vi "zs_newexample.vi"() -> ()   [LabVIEW 2014]
uses:
  <vilib>/regexp/Match Regular Expression.xnode
panel:
  out "错误输出":errorcluster
  out "数据输出":string
  out "standard error":string caption="标准错误"
  out "error out":errorcluster caption="错误输出"
  out "数组":string[][](array[string])
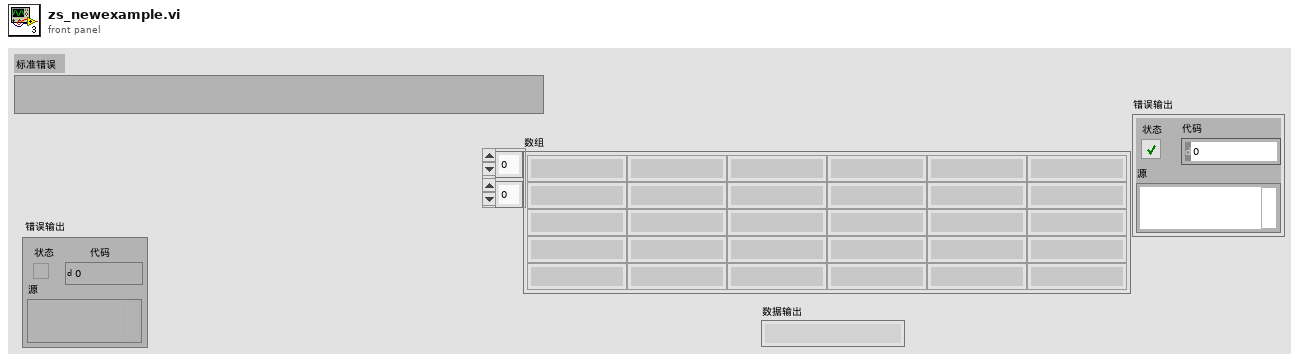
[diagram p1: front panel]
types:
  T1 = enum16{"Standard", "Buffered", "CRLF", "Immediate"}
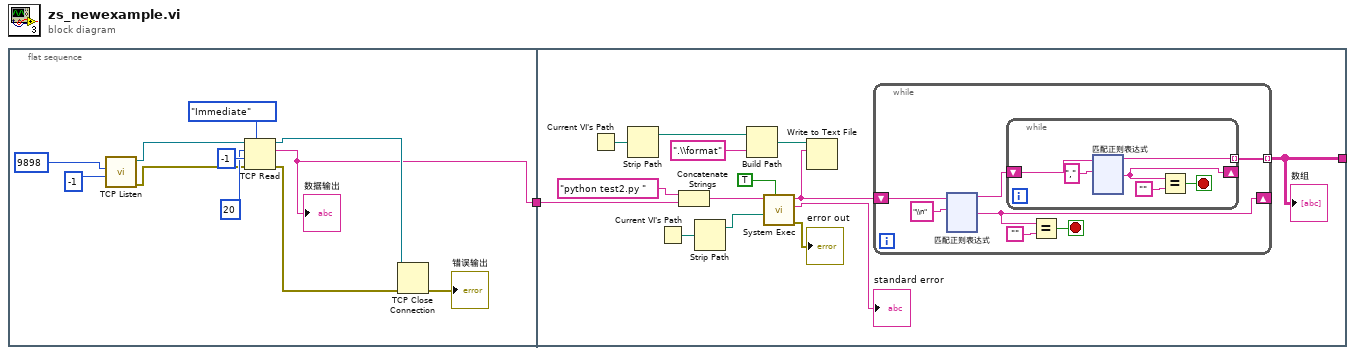
[diagram p0: block diagram]
diagram:
  n1 = flat-sequence {
    tunnel: [w2] -> w1
    tunnel: w1 -> [w19]
    tunnel: [w13] -> _
    frame #0 {
      n2 = call <vilib>:"TCP Listen.vi"("timeout ms (wait forever: -1)"=-1, "port"=u16 9898) -> ("error out"=w3:errorcluster, "connection ID"=w7:refnum<k5>)  [unwired: 5 in, 3 out]
      n3 = TCP Read(connection ID=w7, bytes to read=20 ("读取的字节"), error in (no error)=w3, 7:T1."Immediate" ("模式（标准）"), 9:-1 ("超时毫秒(25000)")) -> (connection ID out=w6:refnum<k5>, data out=w2:string, error out=w11:errorcluster)
      "数据输出" <- w2
      n4 = TCP Close Connection(connection ID=w6, error in (no error)=w11) -> (error out=→"错误输出":errorcluster)  [unwired: 1 in, 1 out]
    }
    frame #1 {
      n5 = Current VI's Path() -> (path=w18:path)
      n6 = Strip Path(path=w18) -> (stripped path=w17:path)  [unwired: 1 out]
      n7 = Current VI's Path() -> (path=w22:path)
      n8 = Concatenate Strings("python test2.py " ("command line"), w19) -> (w20:string)
      n9 = Strip Path(path=w22) -> (stripped path=w23:path)  [unwired: 1 out]
      n10 = Build Path(base path=w17, name or relative path=".\\format" ("名称或相对路径")) -> (appended path=w15:path)
      n11 = call <vilib>:"System Exec.vi"("wait until completion? (T)"=TRUE, "working directory"=w23, "command line"=w20) -> ("error out"=→"error out":errorcluster, "standard error"=→"standard error":string, "standard output"=w14:string)  [unwired: 5 in, 1 out]
      n12 = Write to Text File(file (use dialog)=w15, text=w14) -> ()  [unwired: 2 in, 3 out]
      n13 = while {
        tunnel: [w27] -> w13 mode=indexing
        shift-right: [w31] -> _
        shift-left: w14 -> [w32]
        stop <- w29 stop-if-true
        n14 = xnode "匹配正则表达式"("输入字符串"=w32, "正则表达式"="\\n") -> ("匹配之前"=w28:string, "匹配之后"=w31:string)  [unwired: 4 in, 3 out]
        n15 = while {
          shift-right: [w35] -> _
          shift-left: w28 -> [w39]
          tunnel: [w37] -> w27 mode=indexing
          stop <- w34 stop-if-true
          n16 = xnode "匹配正则表达式"("输入字符串"=w39, "正则表达式"=",") -> ("匹配之前"=w37:string, "匹配之后"=w35:string)  [unwired: 4 in, 3 out]
          n17 = Equal?(x=w35, y="") -> (x = y?=w34:bool)
        }
        n18 = Equal?(x=w31, y="") -> (x = y?=w29:bool)
      }
      "数组" <- w13
    }
  }
